vi "sub_multipart.vi"() -> ()   [LabVIEW 2019]
uses:
  vi.lib/addons/zeromq/socket_type.ctl
  vi.lib/addons/zeromq/socket_options.ctl
  vi.lib/addons/zeromq/zeromq.lvlib
  vi.lib/addons/zeromq/zmq_context.lvclass
  vi.lib/addons/zeromq/zmq_socket.lvclass
panel:
  out "message":string[](array[string])
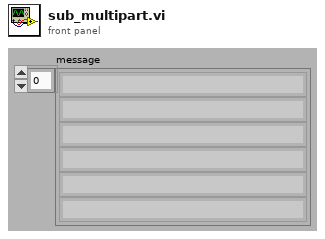
[diagram p1: front panel]
types:
  T1 = typedef "zeromq.lvlib/socket_options.ctl" = enum8{"NONE", "ZMQ_HWM", "<2>", "ZMQ_SWAP", "ZMQ_AFFINITY", "ZMQ_IDENTITY", "ZMQ_SUBSCRIBE", "ZMQ_UNSUBSCRIBE", "ZMQ_RATE", "ZMQ_RECOVERY_IVL", "ZMQ_MCAST_LOOP", "ZMQ_SNDBUF", "ZMQ_RCVBUF", "ZMQ_RCVMORE", "ZMQ_FD", "ZMQ_EVENTS", "ZMQ_TYPE", "ZMQ_LINGER", "ZMQ_RECONNECT_IVL", "ZMQ_BACKLOG", "ZMQ_RECOVERY_IVL_MSEC", "ZMQ_RECONNECT_IVL_MAX", "ZMQ_MAXMSGSIZE", "ZMQ_SNDHWM", "ZMQ_RCVHWM", "ZMQ_MULTICAST_HOPS", "<26>", "ZMQ_RCVTIMEO", "ZMQ_SNDTIMEO", "<29>", "<30>", "ZMQ_IPV4ONLY", "ZMQ_LAST_ENDPOINT", "ZMQ_ROUTER_MANDATORY", "ZMQ_TCP_KEEPALIVE", "ZMQ_TCP_KEEPALIVE_CNT", "ZMQ_TCP_KEEPALIVE_IDLE", "ZMQ_TCP_KEEPALIVE_INTVL", "ZMQ_TCP_ACCEPT_FILTER", "ZMQ_DELAY_ATTACH_ON_CONNECT", "ZMQ_XPUB_VERBOSE"}
  T2 = typedef "zeromq.lvlib/socket_type.ctl" = enum8{"ZMQ_PAIR", "ZMQ_PUB", "ZMQ_SUB", "ZMQ_REQ", "ZMQ_REP", "ZMQ_DEALER", "ZMQ_ROUTER", "ZMQ_PULL", "ZMQ_PUSH", "ZMQ_XPUB", "ZMQ_XSUB"}
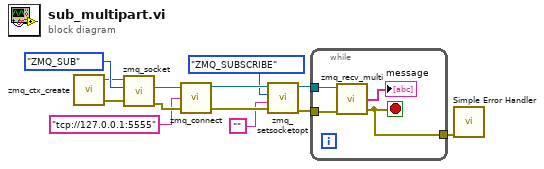
[diagram p0: block diagram]
diagram:
  n1 = call "zmq_ctx_create.vi"() -> ("error out"=w12:errorcluster, "context out"=w1:refnum<class "zmq_context.lvclass">)  [unwired: 4 in]
  n2 = call "zmq_socket.vi"("error in"=w12, "socket type"=socket_type."ZMQ_SUB", "context in"=w1) -> ("error out"=w11:errorcluster, "socket out"=w2:refnum<class "zmq_socket.lvclass">)  [unwired: 2 in, 1 out]
  n3 = call "zmq_connect.vi"("error in"=w11, "endpoint"="tcp://127.0.0.1:5555", "socket in"=w2) -> ("error out"=w9:errorcluster, "socket out"=w10:refnum<class "zmq_socket.lvclass">)  [unwired: 1 in]
  n4 = call "zmq_setsocketopt.vi"("error in"=w9, "value"="", "option"=socket_options."ZMQ_SUBSCRIBE", "socket in"=w10) -> ("error out"=w8:errorcluster, "socket out"=w7:refnum<class "zmq_socket.lvclass">)  [unwired: 2 in]
  n5 = while {
    tunnel: w7 -> [w17]
    tunnel: w8 -> [w15]
    tunnel: [w14] -> w3
    stop <- w14 stop-if-true
    n6 = call "zmq_recv_multi.vi"("error in"=w15, "socket in"=w17) -> ("error out"=w14:errorcluster, "parts"=→"message":string[])  [unwired: 1 in, 1 out]
  }
  n7 = call <vilib>:"Simple Error Handler.vi"("error in (no error)"=w3) -> ()  [unwired: 4 in, 5 out]
